vi "Main Menu 3.1.vi"() -> ()   [LabVIEW 2020]
uses:
  Controls/DataCluster.ctl
  <vilib>/Utility/miscctls.llb/LVCursorListTypeDef.ctl
  Controls/Selector Cases.ctl
panel:
  in  "Settings Button":bool
  in  "Batch Button":bool
  in  "Event & Sensor Select Button":bool
  in  "Add Annotations":bool
  in  "Figures Button":bool
  in  "Help Button":bool
  in  "Extract Button":bool
  in  "NMD Button":bool
  in  "SPARC Button":bool
  out "UI Message":string
  in  "Open Button":bool
  # "Spectral Analysis"
  # "Extras"
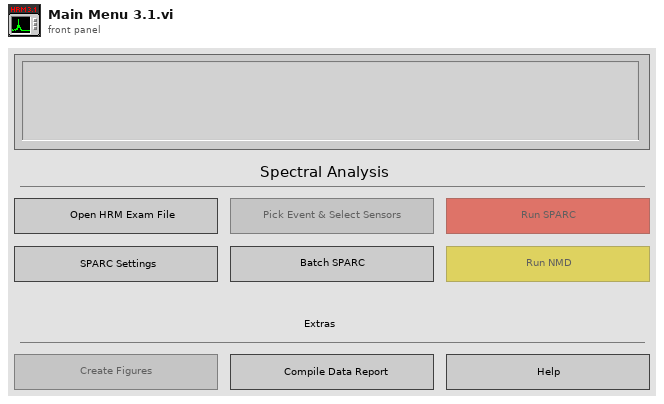
[diagram p1: front panel]
types:
  T1 = typedef "Selector Cases.ctl" = enum16{"Initialize", "Wait", "Open", "Find Segment", "Update Sensor Plots", "Analyze", "Save", "Exit"}
  T2 = cluster{"Add Annotations":refnum<vi>, "Event & Sensor Select Button":refnum<vi>, "SPARC Button":refnum<vi>, "NMD Button":refnum<vi>, "Sleep Mano Button":refnum<vi>, "Spatio Button":refnum<vi>, "Extract Button":refnum<vi>}
  T3 = typedef "DataCluster.ctl" = cluster{"Selected File":path, "Full Text File":string[][], "Data Array":dbl[][], "Times Array":dbl[], "Sensor Array":dbl[], "Subset Array":dbl[][], "Smoothness Values":dbl[], "Sensor Select 1":refnum<vi>, "Sensor Select 2":refnum<vi>, "Sensor Select 3":refnum<vi>, "Sensor Select 4":refnum<vi>, "Start Times":dbl[], "End Times":dbl[], "Cursor List":T4, "Listbox 1":refnum<vi>, "Listbox 2":refnum<vi>, "Listbox 3":refnum<vi>, "Listbox 4":refnum<vi>, "Labels":string[], "Event Array":dbl[][], "Event Names":string[], "Event Times":dbl[], "Save Plot Button":refnum<vi>, "Sensor Plot Refs":refnum<vi>[], "Selected Event (Title)":string, "Upper Cursor":dbl, "Lower Cursor":dbl, "Z Max":dbl, "Z Min":dbl}
  T4 = typedef "LVCursorListTypeDef.ctl" = cluster{"Name":string, "Color":u32, "Style":u8, "Point Style":u8, "Name Visible":bool, "Allow Drag":bool, "Cursor Mode":u32, "Plot":i32, "Index":i32, "Position":cluster{"X":dbl, "Y":dbl}, "X Scale":u32, "Y Scale":u32, "Watch Plots":i32[], "Watch All Plots":bool, "Plot Area":i32, "Label Offset":cluster{"X":dbl, "Y":dbl}}[]
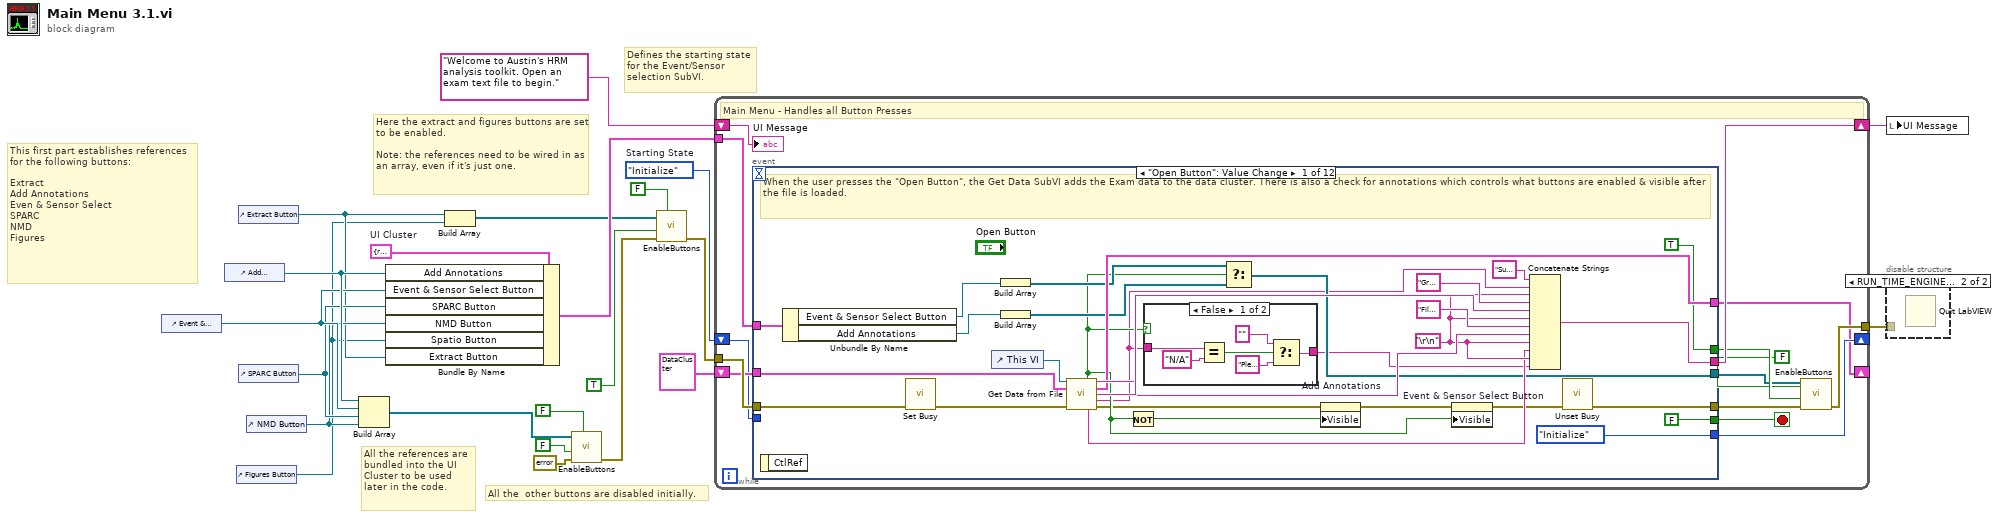
[diagram p0: block diagram]
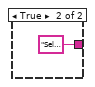
[diagram p3: hidden frame]
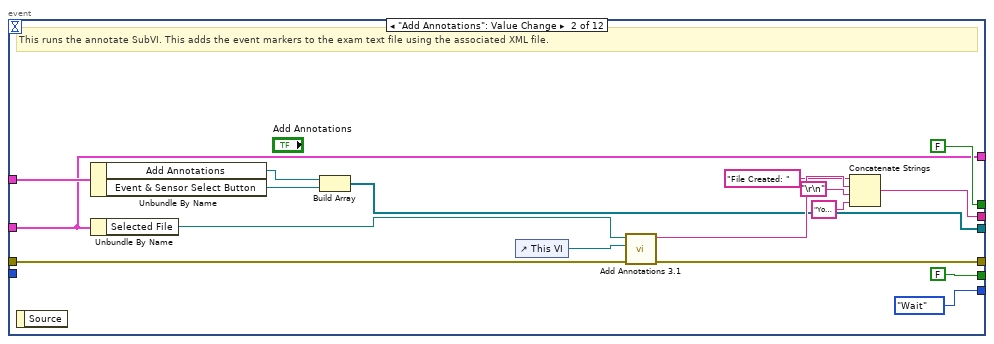
[diagram p4: hidden frame]
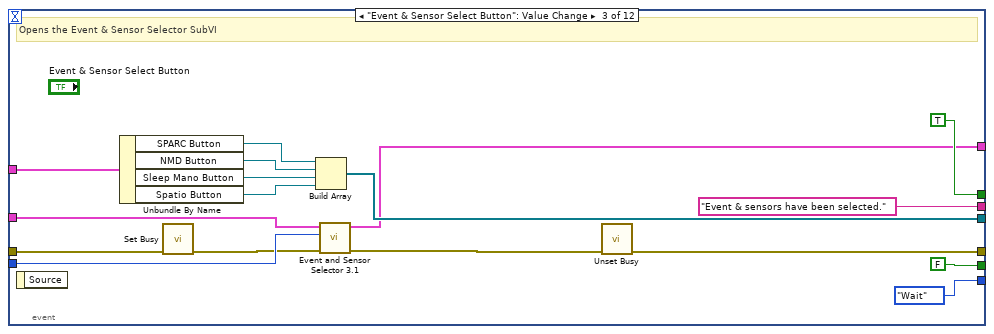
[diagram p5: hidden frame]
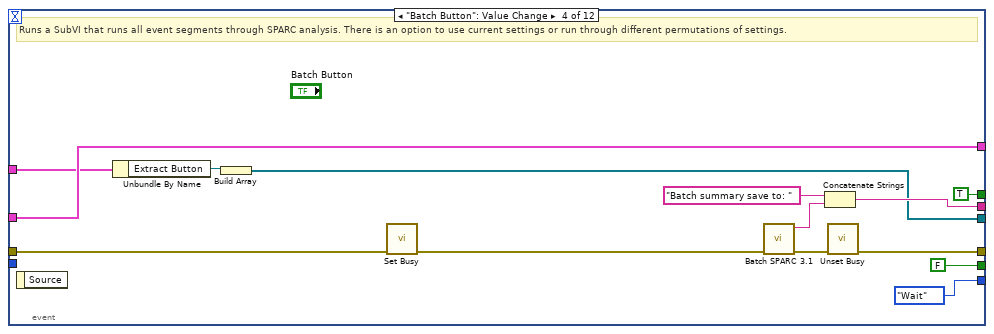
[diagram p6: hidden frame]
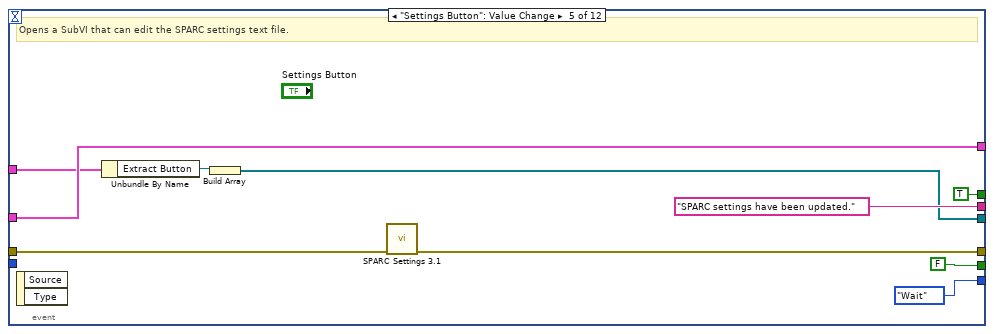
[diagram p7: hidden frame]
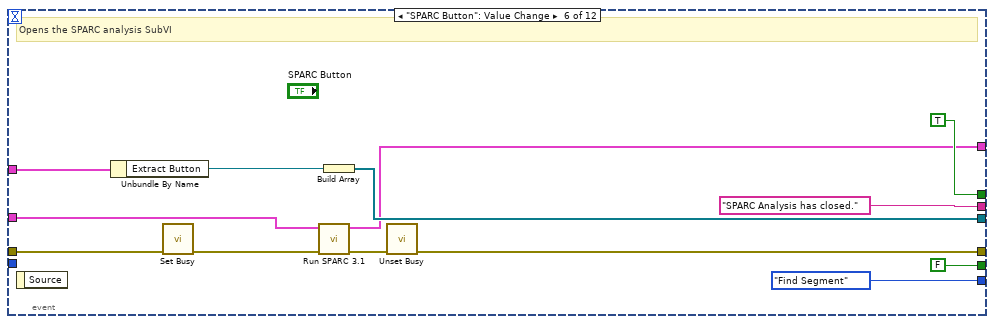
[diagram p8: hidden frame]
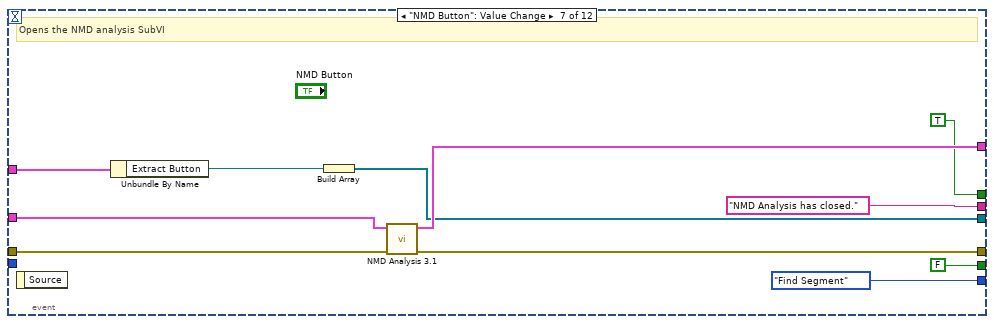
[diagram p9: hidden frame]
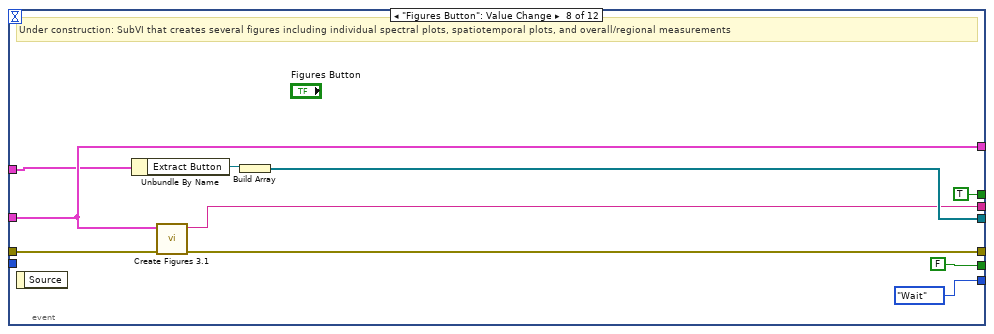
[diagram p10: hidden frame]
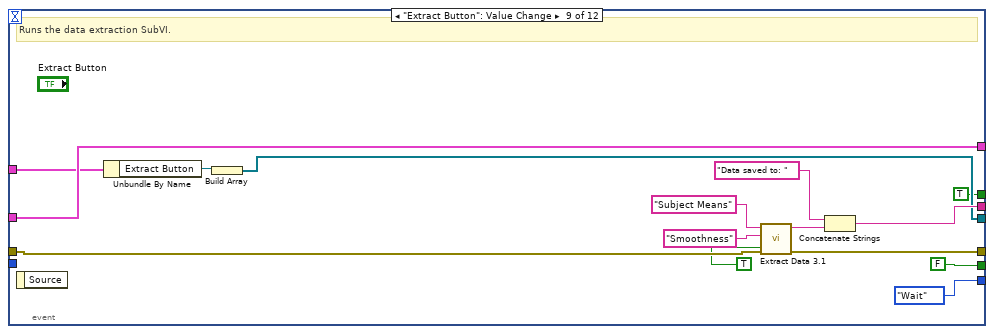
[diagram p11: hidden frame]
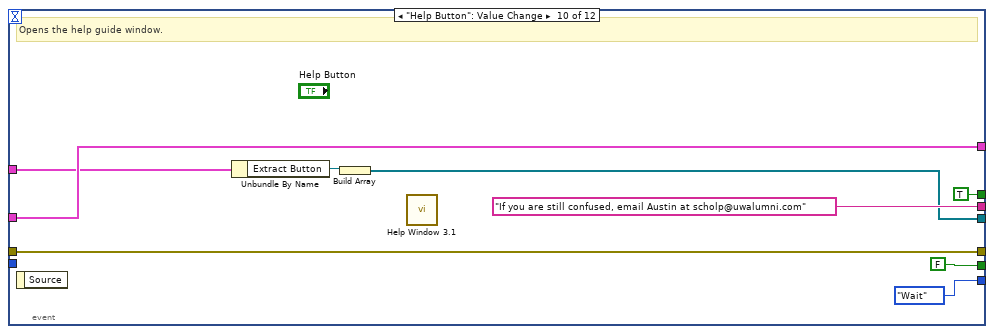
[diagram p12: hidden frame]
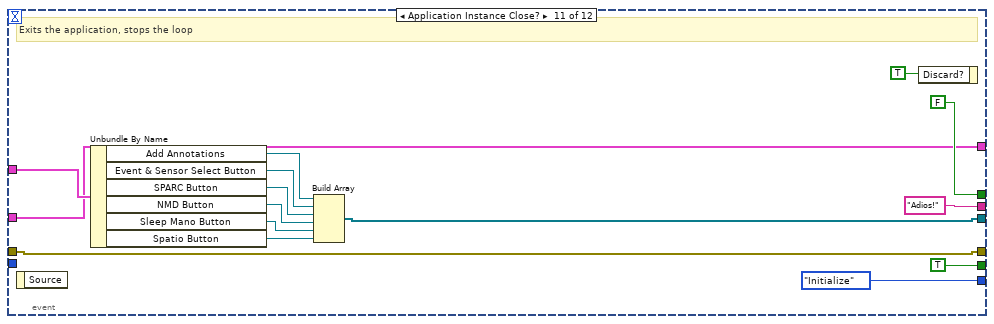
[diagram p13: hidden frame]
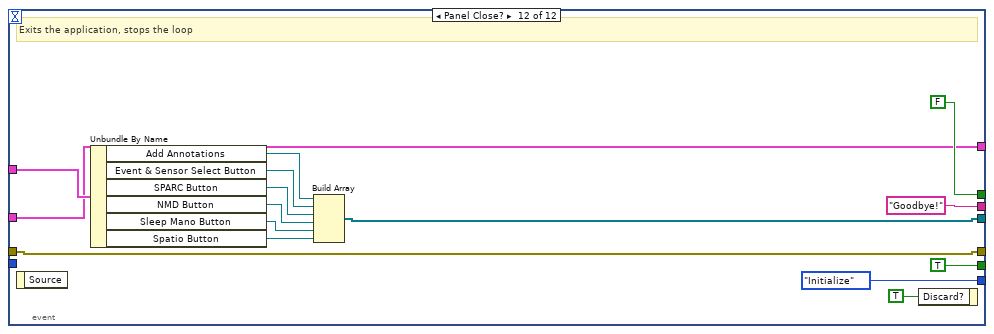
[diagram p14: hidden frame]
diagram:
  w5 = Selector_Cases."Initialize"  # Starting State
  w15 = T2 {"Add Annotations"=refnum, "Event & Sensor Select Button"=refnum, "SPARC Button"=refnum, "NMD Button"=refnum, "Sleep Mano Button"=refnum, "Spatio Button"=refnum, "Extract Button"=refnum}  # UI Cluster
  # "Defines the starting state for the Event/Sensor selection SubVI."
  # "All the references are bundled into the UI Cluster to be used later in the code."
  # "All the  other buttons are disabled initially."
  # "Here the extract and figures buttons are set to be enabled. \n\nNote: the references need to be wired in as an array, even if it's just one."
  # "This first part establishes references for the following buttons:\n\nExtract\nAdd Annotations\nEven & Sensor Select\nSPARC\nNMD\nFigures"
  n1 = control-ref of="Event & Sensor Select Button"() -> (w13:refnum<vi>)
  n2 = control-ref of="Add Annotations"() -> (w14:refnum<vi>)
  n3 = control-ref of="Figures Button"() -> (w1:refnum<vi>)
  n4 = control-ref of="Extract Button"() -> (w4:refnum<vi>)
  n5 = control-ref of="SPARC Button"() -> (w12:refnum<vi>)
  n6 = control-ref of="NMD Button"() -> (w11:refnum<vi>)
  n7 = Build Array "Build Array"(w14, w13, w12, w11) -> (w17:refnum<vi>[])
  n8 = Bundle By Name(cluster=w15, "Add Annotations"=w14, "Event & Sensor Select Button"=w13, "SPARC Button"=w12, "NMD Button"=w11, "Spatio Button"=w1, "Extract Button"=w4) -> (w10:T2)
  n9 = Build Array "Build Array"(w4, w1) -> (w9:refnum<vi>[])
  n10 = call "EnableButtons.vi"("Change Visibility?"=FALSE, "Error In"=errorcluster {"status"=FALSE, "code"=0, "source"=""} ("error in (no error)"), "Enable?"=FALSE, "Button Ref Array"=w17) -> ("Error Out"=w7:errorcluster)  [unwired: 7 in]
  n11 = call "EnableButtons.vi"("Change Visibility?"=FALSE, "Error In"=w7, "Enable?"=TRUE, "Button Ref Array"=w9) -> ("Error Out"=w6:errorcluster)  [unwired: 7 in]
  n12 = while {
    shift-right: [w34] -> w19
    shift-left: "Welcome to Austin's HRM analysis toolkit. Open an exam text file to begin." ("UI Message") -> [w36]
    tunnel: w6 -> [w33]
    tunnel: [w30] -> w21
    shift-right: [w24] -> _
    shift-left: T3 {"Selected File"=path "", "Full Text File"=[], "Data Array"=[], "Times Array"=[], "Sensor Array"=[], "Subset Array"=[], "Smoothness Values"=[], "Sensor Select 1"=refnum, "Sensor Select 2"=refnum, "Sensor Select 3"=refnum, "Sensor Select 4"=refnum, "Start Times"=[], "End Times"=[], "Cursor List"=[{"Name"="Event Marker          ", "Color"=16777200, "Style"=0, "Point Style"=0, "Name Visible"=FALSE, "Allow Drag"=FALSE, "Cursor Mode"=0, "Plot"=0, "Index"=0, "Position"={"X"=4.0, "Y"=1.0}, "X Scale"=0, "Y Scale"=0, "Watch Plots"=[], "Watch All Plots"=FALSE, "Plot Area"=0, "Label Offset"={"X"=-50.0, "Y"=150.0}}, {"Name"="Upper Sensor", "Color"=13816500, "Style"=6, "Point Style"=0, "Name Visible"=FALSE, "Allow Drag"=FALSE, "Cursor Mode"=0, "Plot"=0, "Index"=0, "Position"={"X"=-1.0, "Y"=5.0}, "X Scale"=0, "Y Scale"=0, "Watch Plots"=[], "Watch All Plots"=FALSE, "Plot Area"=0, "Label Offset"={"X"=0.0, "Y"=0.0}}, {"Name"="Lower Sensor", "Color"=13816500, "Style"=6, "Point Style"=0, "Name Visible"=FALSE, "Allow Drag"=FALSE, "Cursor Mode"=0, "Plot"=0, "Index"=0, "Position"={"X"=-1.0, "Y"=30.0}, "X Scale"=0, "Y Scale"=0, "Watch Plots"=[], "Watch All Plots"=FALSE, "Plot Area"=0, "Label Offset"={"X"=0.0, "Y"=0.0}}], "Listbox 1"=refnum, "Listbox 2"=refnum, "Listbox 3"=refnum, "Listbox 4"=refnum, "Labels"=["Why", "is", "this", "still", "not", "built", "into", "Labview?", "This", "is", "shameful."], "Event Array"=[], "Event Names"=[], "Event Times"=[], "Save Plot Button"=refnum, "Sensor Plot Refs"=[], "Selected Event (Title)"="", "Upper Cursor"=0.0, "Lower Cursor"=0.0, "Z Max"=0.0, "Z Min"=0.0} ("Data Cluster") -> [w32]
    tunnel: w10 -> [w28]
    shift-right: [w25] -> _
    shift-left: w5 -> [w26]
    stop <- w35 stop-if-true
    # "Main Menu - Handles all Button Presses"
    n13 = event shown="[0] \"Open Button\": Value Change" {
      selector: _ -> [_ _ _ _ _ _ _ _ _ _ _ _]
      dyn-events: _ -> [_ _ _ _ _ _ _ _ _ _ _ _]
      timeout: _ -> [_ _ _ _ _ _ _ _ _ _ _ _]
      tunnel: [FALSE FALSE FALSE FALSE FALSE FALSE FALSE FALSE FALSE FALSE TRUE TRUE] -> w35
      tunnel: [w63 w84 "Event & sensors have been selected." w118 "SPARC settings have been updated." "SPARC Analysis has closed." "NMD Analysis has closed." w156 w177 "If you are still confused, email Austin at scholp@uwalumni.com" "Adios!" "Goodbye!"] -> w34
      tunnel: w33 -> [w43 w89 w93 w115 w131 w136 w152 w162 w179 w188 w197 w216]
      tunnel: [w45 w88 w91 w113 w130 w137 w151 w161 w178 w188 w197 w216] -> w31
      tunnel: w32 -> [w65 w77 w105 w112 w127 w132 w150 w163 w174 w187 w191 w206]
      tunnel: [w57 w77 w96 w112 w127 w133 w149 w163 w174 w187 w191 w206] -> w24
      tunnel: [TRUE FALSE TRUE TRUE TRUE TRUE TRUE TRUE TRUE TRUE FALSE FALSE] -> w29
      tunnel: w28 -> [w55 w78 w104 w111 w124 w141 w147 w159 w168 w183 w201 w209]
      tunnel: [w52 w81 w99 w109 w123 w139 w146 w158 w167 w182 w192 w208] -> w27
      tunnel: w26 -> [_ _ w97 _ _ _ _ _ _ _ _ _]
      tunnel: [Selector_Cases."Initialize" ("Starting State") Selector_Cases."Wait" ("Starting State") Selector_Cases."Wait" ("Starting State") Selector_Cases."Wait" ("Starting State") Selector_Cases."Wait" ("Starting State") Selector_Cases."Find Segment" ("Starting State") Selector_Cases."Find Segment" ("Starting State") Selector_Cases."Wait" ("Starting State") Selector_Cases."Wait" ("Starting State") Selector_Cases."Wait" ("Starting State") Selector_Cases."Initialize" ("Starting State") Selector_Cases."Initialize" ("Starting State")] -> w25
      event "Open Button": Value Change {
        w54 = "\r\n"
        # "When the user presses the \"Open Button\", the Get Data SubVI adds the Exam data to the data cluster. There is also a check for annotations which controls what buttons are enabled & visible after the file is loaded."
        n14 = event-data() -> ()  [unwired: 1 in, 1 out]
        n15 = Unbundle By Name(w55) -> ("Event & Sensor Select Button"=w48:refnum<vi>, "Add Annotations"=w51:refnum<vi>)
        n16 = call <vilib>:"Set Busy.vi"("error in (no error)"=w43) -> ("error out"=w44:errorcluster)  [unwired: 9 in, 1 out]
        n17 = control-ref of="This VI"() -> (w64:refnum<vi>)
        n18 = Build Array(w48) -> (w50:refnum<vi>[])
        n19 = Build Array(w51) -> (w49:refnum<vi>[])
        n20 = call "Get Data from File.vi"("VI Ref"=w64, "Data Cluster In"=w65, "error in (no error)"=w44) -> ("Has Annotations?"=w41:bool, "File Name"=w58:string, "Data Cluster Out"=w57:T3, "Subject Group"=w60:string, "Subject Number"=w37:string, "Has Annotations"=w53:string, "error out"=w38:errorcluster)  [unwired: 6 in]
        n21 = Not(x=w41) -> (.not. x?=w42:bool)
        n22 = case shown="False" w41 {
          tunnel: [w67 "Select an event and sensors to analyze." ("string")] -> w47
          tunnel: w37 -> [w71 _]
          frame False {
            n23 = Equal?(x=w71, y="N/A") -> (x = y?=w72:bool)
            n24 = Select(t="", s=w72, f="Please add annotations." ("string")) -> (s? t:f=w67:string)
          }
          frame True {
          }
        }
        n25 = Select(t=w50, s=w41, f=w49) -> (s? t:f=w52:refnum<vi>[])
        n26 = property on="Add Annotations" class="Bool"(error in=w38, "Visible"=w42) -> (error out=w39:errorcluster)  [unwired: 1 in, 1 out]
        n27 = property on="Event & Sensor Select Button" class="Bool"(error in=w39, "Visible"=w41) -> (error out=w40:errorcluster)  [unwired: 1 in, 1 out]
        n28 = Concatenate Strings("Subject Number: " ("string"), w37, w54, "Group: " ("string"), w60, w54, "File Opened: " ("UI Message"), w58, w54, w53, w54, w47) -> (w63:string)
        n29 = call <vilib>:"Unset Busy.vi"("error in (no error)"=w40) -> ("error out"=w45:errorcluster)  [unwired: 10 in]
      }
      event "Add Annotations": Value Change {
        # "This runs the annotate SubVI. This adds the event markers to the exam text file using the associated XML file."
        n30 = event-data() -> ()  [unwired: 1 in, 1 out]
        n31 = Unbundle By Name(w78) -> ("Add Annotations"=w79:refnum<vi>, "Event & Sensor Select Button"=w80:refnum<vi>)
        n32 = Unbundle By Name(w77) -> ("Selected File"=w87:path)
        n33 = Build Array(w79, w80) -> (w81:refnum<vi>[])
        n34 = control-ref of="This VI"() -> (w86:refnum<vi>)
        n35 = call "Add Annotations 3.1.vi"("error in"=w89, "VI reference"=w86, "File to be Annotated"=w87) -> ("error out"=w88:errorcluster, "Annotated File"=w85:string)  [unwired: 7 in]
        n36 = Concatenate Strings("File Created: " ("string"), w85, "\r\n", "You have to open the new annotated file." ("string")) -> (w84:string)
      }
      event "Event & Sensor Select Button": Value Change {
        # "Opens the Event & Sensor Selector SubVI"
        n37 = event-data() -> ()  [unwired: 1 in, 1 out]
        n38 = Unbundle By Name(w104) -> ("SPARC Button"=w103:refnum<vi>, "NMD Button"=w102:refnum<vi>, "Sleep Mano Button"=w101:refnum<vi>, "Spatio Button"=w100:refnum<vi>)
        n39 = call <vilib>:"Set Busy.vi"("error in (no error)"=w93) -> ("error out"=w94:errorcluster)  [unwired: 9 in, 1 out]
        n40 = Build Array(w103, w102, w101, w100) -> (w99:refnum<vi>[])
        n41 = call "Event and Sensor Selector 3.1.vi"("error in"=w94, "Starting State"=w97, "Data Cluster In"=w105) -> ("error out"=w92:errorcluster, "Data Cluster Out"=w96:T3)  [unwired: 7 in]
        n42 = call <vilib>:"Unset Busy.vi"("error in (no error)"=w92) -> ("error out"=w91:errorcluster)  [unwired: 10 in]
      }
      event "Batch Button": Value Change {
        # "Runs a SubVI that runs all event segments through SPARC analysis. There is an option to use current settings or run through different permutations of settings."
        n43 = event-data() -> ()  [unwired: 1 in, 1 out]
        n44 = Unbundle By Name(w111) -> ("Extract Button"=w110:refnum<vi>)
        n45 = Build Array(w110) -> (w109:refnum<vi>[])
        n46 = call <vilib>:"Set Busy.vi"("error in (no error)"=w115) -> ("error out"=w116:errorcluster)  [unwired: 9 in, 1 out]
        n47 = call "Batch SPARC 3.1.vi"("Error In"=w116) -> ("Error Out"=w114:errorcluster, "Saved Path"=w119:string)  [unwired: 9 in]
        n48 = Concatenate Strings("Batch summary save to: ", w119) -> (w118:string)
        n49 = call <vilib>:"Unset Busy.vi"("error in (no error)"=w114) -> ("error out"=w113:errorcluster)  [unwired: 10 in]
      }
      event "Settings Button": Value Change {
        # "Opens a SubVI that can edit the SPARC settings text file."
        n50 = event-data() -> ()  [unwired: 1 in, 2 out]
        n51 = Unbundle By Name(w124) -> ("Extract Button"=w125:refnum<vi>)
        n52 = Build Array(w125) -> (w123:refnum<vi>[])
        n53 = call "SPARC Settings 3.1.vi"("error in (no error)"=w131) -> ("error out"=w130:errorcluster)  [unwired: 10 in]
      }
      event "SPARC Button": Value Change {
        # "Opens the SPARC analysis SubVI"
        n54 = event-data() -> ()  [unwired: 1 in, 1 out]
        n55 = Unbundle By Name(w141) -> ("Extract Button"=w140:refnum<vi>)
        n56 = call <vilib>:"Set Busy.vi"("error in (no error)"=w136) -> ("error out"=w135:errorcluster)  [unwired: 9 in, 1 out]
        n57 = call "Run SPARC 3.1.vi"("error in (no error)"=w135, "Data Cluster In"=w132) -> ("error out"=w134:errorcluster, "Data Cluster Out"=w133:T3)  [unwired: 8 in]
        n58 = Build Array(w140) -> (w139:refnum<vi>[])
        n59 = call <vilib>:"Unset Busy.vi"("error in (no error)"=w134) -> ("error out"=w137:errorcluster)  [unwired: 10 in]
      }
      event "NMD Button": Value Change {
        # "Opens the NMD analysis SubVI"
        n60 = event-data() -> ()  [unwired: 1 in, 1 out]
        n61 = Unbundle By Name(w147) -> ("Extract Button"=w148:refnum<vi>)
        n62 = Build Array(w148) -> (w146:refnum<vi>[])
        n63 = call "NMD Analysis 3.1.vi"("error in (no error)"=w152, "Data Cluster In"=w150) -> ("error out"=w151:errorcluster, "Data Cluster Out"=w149:T3)  [unwired: 8 in]
      }
      event "Figures Button": Value Change {
        # "Under construction: SubVI that creates several figures including individual spectral plots, spatiotemporal plots, and overall/regional measurements"
        n64 = event-data() -> ()  [unwired: 1 in, 1 out]
        n65 = Unbundle By Name(w159) -> ("Extract Button"=w160:refnum<vi>)
        n66 = call "Create Figures 3.1.vi"("Error In"=w162, "Data Cluster"=w163) -> ("Error Out"=w161:errorcluster, "Message"=w156:string)  [unwired: 8 in]
        n67 = Build Array(w160) -> (w158:refnum<vi>[])
      }
      event "Extract Button": Value Change {
        # "Runs the data extraction SubVI."
        n68 = event-data() -> ()  [unwired: 1 in, 1 out]
        n69 = Unbundle By Name(w168) -> ("Extract Button"=w169:refnum<vi>)
        n70 = Build Array(w169) -> (w167:refnum<vi>[])
        n71 = call "Extract Data 3.1.vi"("Single/Permutations"=TRUE, "Error In"=w179, "File Search Phrase"="Smoothness", "Summary File Title"="Subject Means") -> ("error out"=w178:errorcluster, "Saved Path"=w175:string)  [unwired: 6 in]
        n72 = Concatenate Strings("Data saved to: " ("string"), w175) -> (w177:string)
      }
      event "Help Button": Value Change {
        # "Opens the help guide window."
        n73 = event-data() -> ()  [unwired: 1 in, 1 out]
        n74 = Unbundle By Name(w183) -> ("Extract Button"=w184:refnum<vi>)
        n75 = Build Array(w184) -> (w182:refnum<vi>[])
        n76 = call "Help Window 3.1.vi"() -> ()  [unwired: 12 in]
      }
      event Application Instance Close? {
        # "Exits the application, stops the loop"
        n77 = event-data() -> ()  [unwired: 1 in, 1 out]
        n78 = Unbundle By Name(w201) -> ("Add Annotations"=w200:refnum<vi>, "Event & Sensor Select Button"=w199:refnum<vi>, "SPARC Button"=w196:refnum<vi>, "NMD Button"=w195:refnum<vi>, "Sleep Mano Button"=w194:refnum<vi>, "Spatio Button"=w193:refnum<vi>)
        n79 = Build Array(w200, w199, w196, w195, w194, w193) -> (w192:refnum<vi>[])
        n80 = event-data("Discard?"=TRUE) -> ()  [unwired: 1 in, 1 out]
      }
      event Panel Close? {
        # "Exits the application, stops the loop"
        n81 = event-data() -> ()  [unwired: 1 in, 1 out]
        n82 = Unbundle By Name(w209) -> ("Add Annotations"=w215:refnum<vi>, "Event & Sensor Select Button"=w214:refnum<vi>, "SPARC Button"=w213:refnum<vi>, "NMD Button"=w212:refnum<vi>, "Sleep Mano Button"=w211:refnum<vi>, "Spatio Button"=w210:refnum<vi>)
        n83 = Build Array(w215, w214, w213, w212, w211, w210) -> (w208:refnum<vi>[])
        n84 = event-data("Discard?"=TRUE) -> ()  [unwired: 1 in, 1 out]
      }
    }
    n85 = call "EnableButtons.vi"("Change Visibility?"=FALSE, "Error In"=w31, "Enable?"=w29, "Button Ref Array"=w27) -> ("Error Out"=w30:errorcluster)  [unwired: 7 in]
    "UI Message" <- w36
  }
  n86 = local write "UI Message"(w19) -> ()
  n87 = disable-structure shown="RUN_TIME_ENGINE==True" {
    disable-tunnel: w21 -> [_ _]
    frame condition #0 (active) {
    }
    frame condition #1 {
      n88 = Quit LabVIEW() -> ()  [unwired: 1 in]
    }
  }
